vi "Read Service Settings File.vi"(8 "error in (no error)":errorcluster) -> (0 "error out":errorcluster, 3 "service settings":T1)   [LabVIEW 2021, in "AudioGenUtility.lvlib"]
uses:
  controls/service settings.ctl
  AudioGenUtility.lvlib
  controls/AudioGenTypeDefs.lvlib
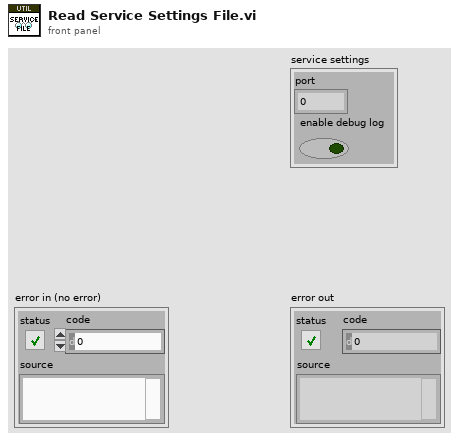
[diagram p1: front panel]
types:
  T1 = typedef "AudioGenTypeDefs.lvlib/service settings.ctl" = cluster{"port":u32, "enable debug log":bool}
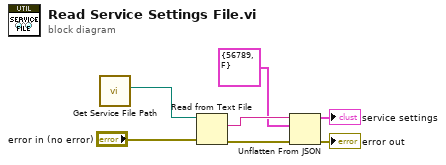
[diagram p0: block diagram]
diagram:
  n1 = call "Get Service File Path.vi"() -> ("service setting file"=w7:path)  [unwired: 11 in]
  n2 = Read from Text File(file (use dialog)=w7, error in="error in (no error)") -> (text=w4:string, error out=w5:errorcluster)  [unwired: 2 in, 2 out]
  n3 = Unflatten From JSON(JSON string=w4, type and defaults=T1 {"port"=56789, "enable debug log"=FALSE} ("service settings"), error in (no error)=w5) -> (value=→"service settings":T1, error out=→"error out":errorcluster)  [unwired: 4 in]
